vi "LOT_System_Setup.vi"(2 "CFG File Path":string) -> (1 "Error Code":i32)   [LabVIEW 2023]
uses:
  SN19523/LOThw/LOThw64.dll
panel:
  out "Initialise System":i32
  out "Build System Model":i32
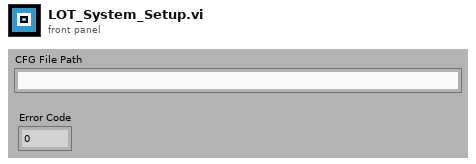
[diagram p1: front panel]
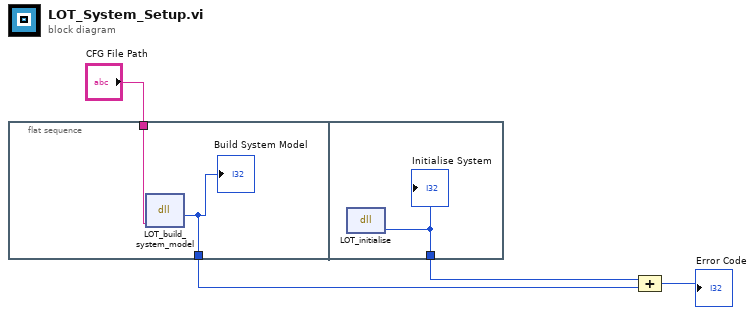
[diagram p0: block diagram]
diagram:
  n1 = flat-sequence {
    tunnel: "CFG File Path" -> [w6]
    tunnel: [w5] -> w2
    tunnel: [w7] -> w3
    frame #0 {
      n2 = dll-call lib="E:/Old PC/desktop/Sensitive EQE Stuff/S-EQE (YJ)/LOT/SN19523/LOThw/LOThw64.dll" fn="LOT_build_system_model"("cfgfile"=w6) -> ("return type"=w5:i32)  [unwired: 4 in, 2 out]
      "Build System Model" <- w5
    }
    frame #1 {
      n3 = dll-call lib="E:/Old PC/desktop/Sensitive EQE Stuff/S-EQE (YJ)/LOT/SN19523/LOThw/LOThw64.dll" fn="LOT_initialise"() -> ("return type"=w7:i16)  [unwired: 3 in, 2 out]
      "Initialise System" <- w7
    }
  }
  n4 = Compound Arithmetic op=ADD(w3, w2) -> (→"Error Code":i32)
